vi "Password Authentication.vi"() -> ()   [LabVIEW 2018]
doc: "Logs into a remote SSH server using a username and password. This is arguably the least secure form of authentication."
uses:
  Toolkit/Session/API/Typedefs/Host Key Hash Types.ctl
  Toolkit/SSH/SSH.lvclass
  Toolkit/Session/Session.lvclass
panel:
  out "Remote Host Key Type":string
  out "Remote Host Key":string
  out "Remote Fingerprint Hash":string
  out "Authenticated":bool
  in  "Remote SSH Server":string
  in  "Password":string
  in  "Username":string
  # "Overview: Demonstrates transferring, or uploading, a local file to a remote SSH server, similar to the SCP command line utility\nInstructions:\n1. Enter the IP address or host name of the remote SSH server. This can be a CompactRIO (cRIO) running the National Instruments Linux Real-Time (NI Linux RT) operating system with the Enable Secure Shell Server (sshd) checkbox checked. \n2. Enter a username. If using a cRIO with a default configuration, then the username is \"admin\".\n3. Enter a password for the username. If using a cRIO with a default configuration, then the password is blank (empty).\n4. Run this VI."
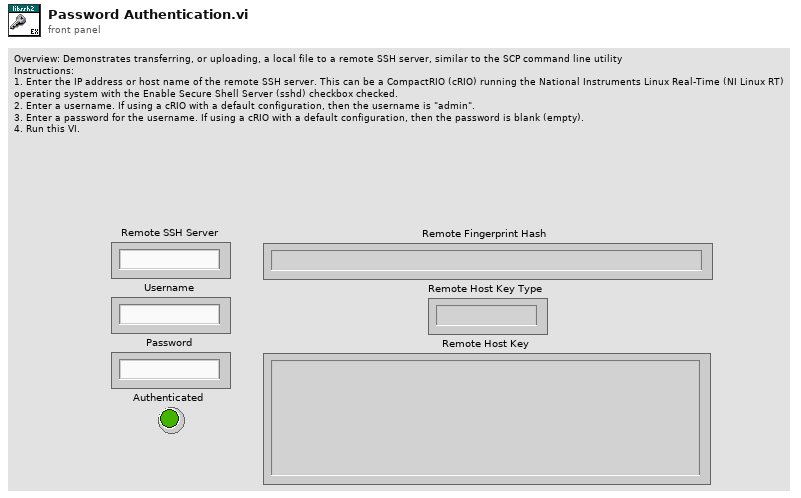
[diagram p1: front panel]
types:
  T1 = typedef "Toolkit.lvlib/Session.lvclass/Host Key Hash Types.ctl" = i32
  T2 = typedef "Toolkit.lvlib/Session.lvclass/Host Key Types.ctl" = i32
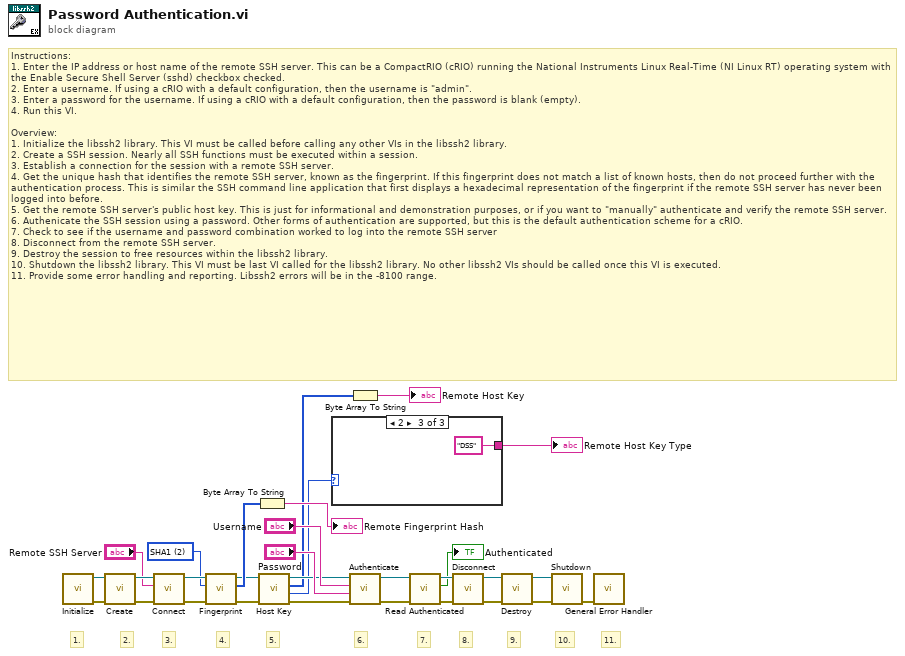
[diagram p0: block diagram]
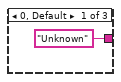
[diagram p2: hidden frame]
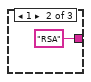
[diagram p3: hidden frame]
diagram:
  w11 = T1 2 items=["MD5"=1, "SHA1"=2] ("Type")
  # "11."
  # "10."
  # "9."
  # "8."
  # "7."
  # "6."
  # "5."
  # "4."
  # "3."
  # "2."
  # "1."
  # "Instructions:\n1. Enter the IP address or host name of the remote SSH server. This can be a CompactRIO (cRIO) running the National Instruments Linux Real-Time (NI Linux RT) operating system with the Enable Secure Shell Server (sshd) checkbox checked. \n2. Enter a username. If using a cRIO with a default configuration, then the username is \"admin\".\n3. Enter a password for the username. If using a cRIO with a default configuration, then the password is blank (empty).\n4. Run this VI.\n\nOverview:\n1. Initialize the libssh2 library. This VI must be called before calling any other VIs in the libssh2 library.\n2. Create a SSH session. Nearly all SSH functions must be executed within a session.\n3. Establish a connection for the session with a remote SSH server.\n4. Get the unique hash that identifies the remote SSH server, known as the fingerprint. If this fingerprint does not match a list of known hosts, then do not proceed further with the authentication process. This is similar the SSH command line application that first displays a hexadecimal representation of the fingerprint if the remote SSH server has never been logged into before.\n5. Get the remote SSH server's public host key. This is just for informational and demonstration purposes, or if you want to \"manually\" authenticate and verify the remote SSH server.\n6. Authenicate the SSH session using a password. Other forms of authentication are supported, but this is the default authentication scheme for a cRIO. \n7. Check to see if the username and password combination worked to log into the remote SSH server\n8. Disconnect from the remote SSH server.\n9. Destroy the session to free resources within the libssh2 library.\n10. Shutdown the libssh2 library. This VI must be last VI called for the libssh2 library. No other libssh2 VIs should be called once this VI is executed.\n11. Provide some error handling and reporting. Libssh2 errors will be in the -8100 range."
  n1 = call "Initialize.vi"() -> ("Error Out"=w29:errorcluster, "SSH"=w30:refnum<class "SSH.lvclass">)  [unwired: 10 in]
  n2 = call "Create.vi"("Error In"=w29, "SSH"=w30) -> ("Error Out"=w27:errorcluster, "Sesssion"=w28:refnum<class "Session.lvclass">)  [unwired: 8 in]
  n3 = call "Connect.vi"("Error In"=w27, "Address"="Remote SSH Server", "Session In"=w28) -> ("Error Out"=w12:errorcluster, "Sesssion Out"=w13:refnum<class "Session.lvclass">)  [unwired: 7 in]
  n4 = call "Fingerprint.vi"("Error In"=w12, "Type"=w11, "Session In"=w13) -> ("Error Out"=w7:errorcluster, "Fingerprint"=w10:u8[], "Sesssion Out"=w8:refnum<class "Session.lvclass">)  [unwired: 6 in]
  n5 = Byte Array To String(unsigned byte array=w10) -> (string=→"Remote Fingerprint Hash":string)
  n6 = call "Host Key.vi"("Error In"=w7, "Session In"=w8) -> ("Error Out"=w6:errorcluster, "Type"=w2:T2, "Host Key"=w4:u8[], "Sesssion Out"=w5:refnum<class "Session.lvclass">)  [unwired: 6 in]
  n7 = case shown="2" w2 {
    tunnel: ["Unknown" "RSA" "DSS"] -> w1
    frame 0, Default {
    }
    frame 1 {
    }
    frame 2 {
    }
  }
  "Remote Host Key Type" <- w1
  n8 = Byte Array To String(unsigned byte array=w4) -> (string=→"Remote Host Key":string)
  n9 = call-poly "Authenticate.vi"("Error In"=w6, "Password"="Password", "Username"="Username", "Session In"=w5) -> ("Error Out"=w18:errorcluster, "Sesssion Out"=w17:refnum<class "Session.lvclass">)  [unwired: 6 in]
  n10 = call "Read Authenticated.vi"("Error In"=w18, "Session In"=w17) -> ("Error Out"=w16:errorcluster, "Authenticated"=→"Authenticated":bool, "Sesssion Out"=w15:refnum<class "Session.lvclass">)  [unwired: 7 in]
  n11 = call "Disconnect.vi"("Error In"=w16, "Session In"=w15) -> ("Error Out"=w22:errorcluster, "Sesssion Out"=w23:refnum<class "Session.lvclass">)  [unwired: 8 in]
  n12 = call "Destroy.vi"("Error In"=w22, "Session"=w23) -> ("Error Out"=w20:errorcluster, "SSH"=w21:refnum<class "SSH.lvclass">)  [unwired: 8 in]
  n13 = call "Shutdown.vi"("Error In"=w20, "SSH"=w21) -> ("Error Out"=w19:errorcluster)  [unwired: 9 in]
  n14 = call <vilib>:"General Error Handler.vi"("error in (no error)"=w19) -> ()  [unwired: 10 in, 5 out]
